vi "Config Logging Readings.vi"(0 "VISA resource name":refnum<visa-resource-name>, 5 "Reading Number (1)":dbl=1.0 min=1.0 max=8.0 step=1.0, 7 "Input to Log (1)":dbl=1.0 min=1.0 max=8.0 step=1.0, 9 "Data Source (0:Kelvin)":u16(ring) items=["Kelvin", "Celsius", "Sensor Units", "Linear Data"], 11 "error in (no error)":errorcluster) -> (4 "VISA resource name out":refnum<visa-resource-name>, 15 "error out":errorcluster)   [LabVIEW 2012, in "Lake Shore Cryotronics 218.lvlib"]
doc: "This VI configures logging parameters that apply to individual readings stored."
uses:
  <instrlib>/Lake Shore Cryotronics 218/Lake Shore Cryotronics 218.lvlib
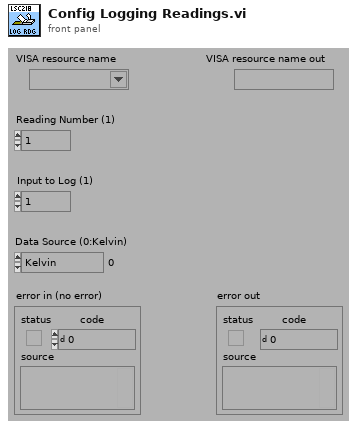
[diagram p1: front panel]
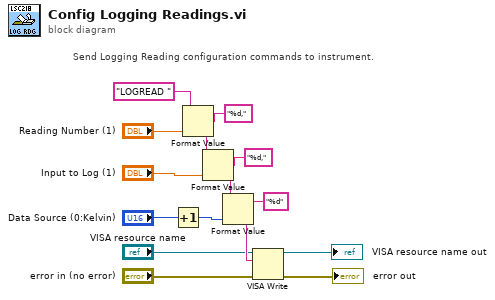
[diagram p0: block diagram]
diagram:
  # "Send Logging Reading configuration commands to instrument."
  n1 = Increment(x="Data Source (0:Kelvin)") -> (x+1=w5:u16)
  n2 = Format Value(string ("")="LOGREAD ", format string="%d,", value (0)="Reading Number (1)") -> (output string=w7:string)
  n3 = Format Value(string ("")=w7, format string="%d,", value (0)="Input to Log (1)") -> (output string=w11:string)
  n4 = Format Value(string ("")=w11, format string="%d", value (0)=w5) -> (output string=w6:string)
  n5 = VISA Write(VISA resource name="VISA resource name", write buffer=w6, error in (no error)="error in (no error)") -> (VISA resource name out=→"VISA resource name out":refnum<visa-resource-name>, error out=→"error out":errorcluster)  [unwired: 1 out]
